vi "zad4.vi"() -> ()   [LabVIEW 2017]
panel:
  out "3":cluster{"1":bool, "2":bool, "3":bool}
  out "4":cluster{"1":bool, "2":bool, "3":bool}
  out "1":cluster{"1":bool, "2":bool, "3":bool}
  in  "Tryb awaryjny":bool
  in  "stop":bool
  out "2":cluster{"1":bool, "2":bool, "3":bool}
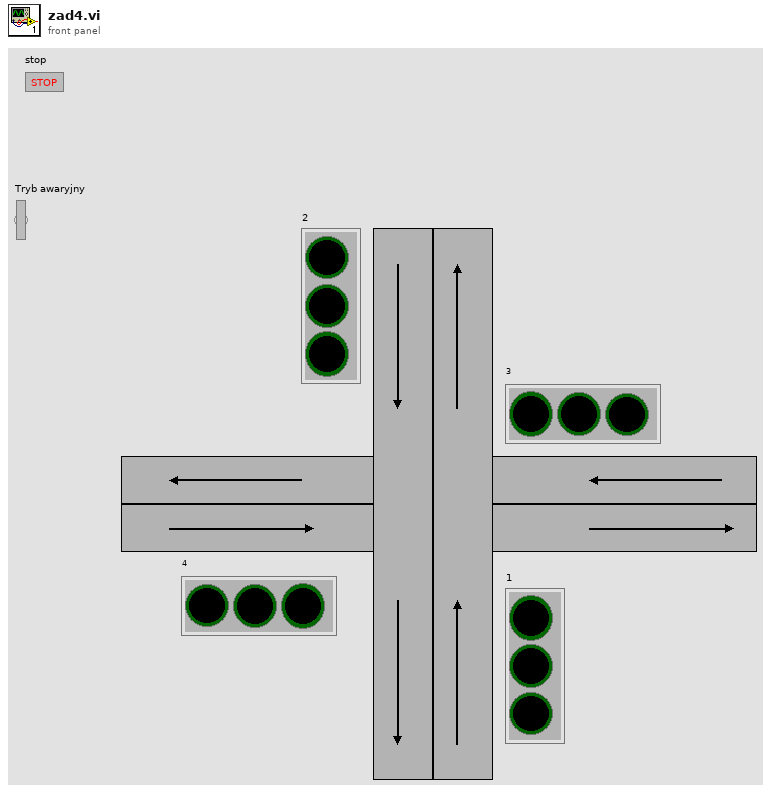
[diagram p1: front panel]
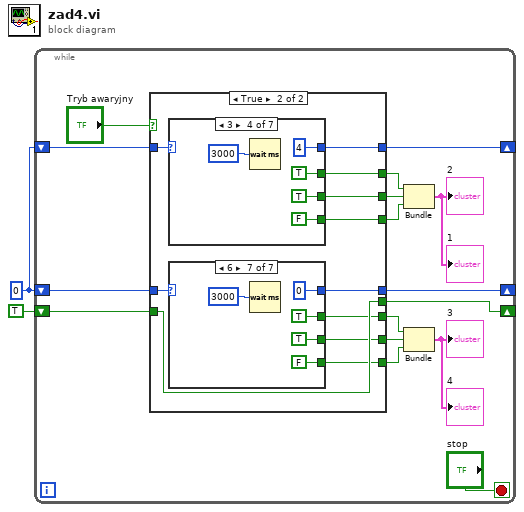
[diagram p0: block diagram]
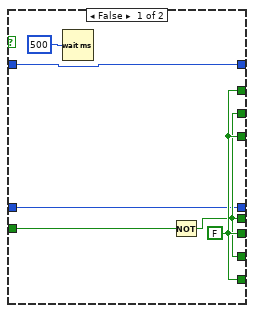
[diagram p2: hidden frame]
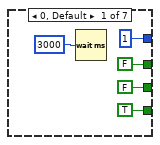
[diagram p3: hidden frame]
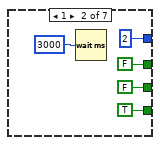
[diagram p4: hidden frame]
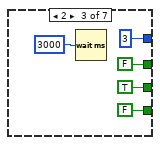
[diagram p5: hidden frame]
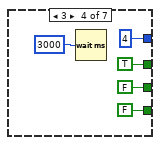
[diagram p6: hidden frame]
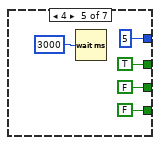
[diagram p7: hidden frame]
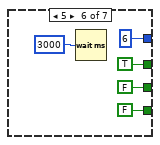
[diagram p8: hidden frame]
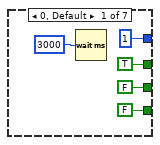
[diagram p9: hidden frame]
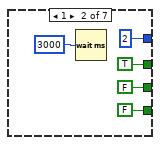
[diagram p10: hidden frame]
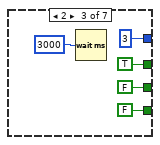
[diagram p11: hidden frame]
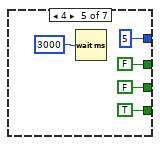
[diagram p12: hidden frame]
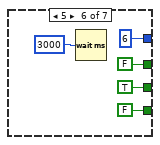
[diagram p13: hidden frame]
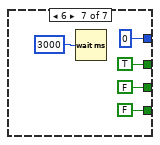
[diagram p14: hidden frame]
diagram:
  w1 = 0
  n1 = while {
    shift-right: [w14] -> _
    shift-left: w1 -> [w3]
    shift-right: [w11] -> _
    shift-left: TRUE ("2") -> [w12]
    shift-right: [w5] -> _
    shift-left: w1 -> [w4]
    stop <- "stop" stop-if-true
    n2 = case shown="True" "Tryb awaryjny" {
      tunnel: [w21 w35] -> w18
      tunnel: [w22 w34] -> w17
      tunnel: [w22 w33] -> w16
      tunnel: [w20 w32] -> w14
      tunnel: [w21 w31] -> w11
      tunnel: w12 -> [w23 w31]
      tunnel: [w21 w29] -> w8
      tunnel: [w22 w28] -> w9
      tunnel: [w22 w30] -> w10
      tunnel: [w19 w27] -> w5
      tunnel: w4 -> [w19 w26]
      tunnel: w3 -> [w20 w25]
      frame False {
        w22 = FALSE ("1")
        n3 = Wait (ms)(milliseconds to wait=500) -> ()  [unwired: 1 out]
        n4 = Not(x=w23) -> (.not. x?=w21:bool)
      }
      frame True {
        n5 = case shown="3" w25 {
          tunnel: [FALSE ("2") FALSE ("2") FALSE ("2") TRUE ("2") FALSE ("2") TRUE ("2") FALSE ("2")] -> w35
          tunnel: [FALSE ("3") FALSE ("3") FALSE ("3") FALSE ("3") TRUE ("3") FALSE ("3") FALSE ("3")] -> w34
          tunnel: [TRUE ("1") TRUE ("1") TRUE ("1") TRUE ("1") FALSE ("1") FALSE ("1") TRUE ("1")] -> w33
          tunnel: [1 2 3 4 5 6 0] -> w32
          frame 0, Default {
            n6 = Wait (ms)(milliseconds to wait=3000) -> ()  [unwired: 1 out]
          }
          frame 1 {
            n7 = Wait (ms)(milliseconds to wait=3000) -> ()  [unwired: 1 out]
          }
          frame 2 {
            n8 = Wait (ms)(milliseconds to wait=3000) -> ()  [unwired: 1 out]
          }
          frame 3 {
            n9 = Wait (ms)(milliseconds to wait=3000) -> ()  [unwired: 1 out]
          }
          frame 4 {
            n10 = Wait (ms)(milliseconds to wait=3000) -> ()  [unwired: 1 out]
          }
          frame 5 {
            n11 = Wait (ms)(milliseconds to wait=3000) -> ()  [unwired: 1 out]
          }
          frame 6 {
            n12 = Wait (ms)(milliseconds to wait=3000) -> ()  [unwired: 1 out]
          }
        }
        n13 = case shown="6" w26 {
          tunnel: [FALSE ("2") FALSE ("2") TRUE ("2") FALSE ("2") FALSE ("2") FALSE ("2") TRUE ("2")] -> w29
          tunnel: [TRUE ("3") TRUE ("3") FALSE ("3") FALSE ("3") FALSE ("3") FALSE ("3") FALSE ("3")] -> w30
          tunnel: [FALSE ("1") FALSE ("1") FALSE ("1") TRUE ("1") TRUE ("1") TRUE ("1") TRUE ("1")] -> w28
          tunnel: [1 2 3 4 5 6 0] -> w27
          frame 0, Default {
            n14 = Wait (ms)(milliseconds to wait=3000) -> ()  [unwired: 1 out]
          }
          frame 1 {
            n15 = Wait (ms)(milliseconds to wait=3000) -> ()  [unwired: 1 out]
          }
          frame 2 {
            n16 = Wait (ms)(milliseconds to wait=3000) -> ()  [unwired: 1 out]
          }
          frame 3 {
            n17 = Wait (ms)(milliseconds to wait=3000) -> ()  [unwired: 1 out]
          }
          frame 4 {
            n18 = Wait (ms)(milliseconds to wait=3000) -> ()  [unwired: 1 out]
          }
          frame 5 {
            n19 = Wait (ms)(milliseconds to wait=3000) -> ()  [unwired: 1 out]
          }
          frame 6 {
            n20 = Wait (ms)(milliseconds to wait=3000) -> ()  [unwired: 1 out]
          }
        }
      }
    }
    n21 = Bundle("1"=w16, "2"=w18, "3"=w17) -> (→"2" →"1":cluster{"1":bool, "2":bool, "3":bool})  [unwired: 1 in]
    n22 = Bundle("1"=w9, "2"=w8, "3"=w10) -> (→"4" →"3":cluster{"1":bool, "2":bool, "3":bool})  [unwired: 1 in]
  }
